vi "Unbundle.vi"(11 "Multi Instrument Wrapper Msg in":refnum<class "Multi Instrument Wrapper Msg.lvclass">) -> (0 "Aquirer Indices":i32[](array[numeric]), 1 "Aquirer":T1[](array[typedef]), 2 "Enqueue Locks":T2[](array[typedef]), 3 "Msg":refnum<class "Multi Instrument Msg.lvclass">)   [LabVIEW 2020, in "Instrument Handler.lvlib" / "Multi Instrument Wrapper Msg.lvclass"]
doc: "Unbundle all the private data from the Msg."
uses:
  Multi Instrument Wrapper Msg.lvclass
  Multi Instrument Msg/Multi Instrument Msg.lvclass
  Controls/Ctl_AquirerRefnum.ctl
  Multi Instrument Wrapper Msg.lvclass/Multi Instrument Wrapper Msg.ctl
  Instrument Handler.lvlib
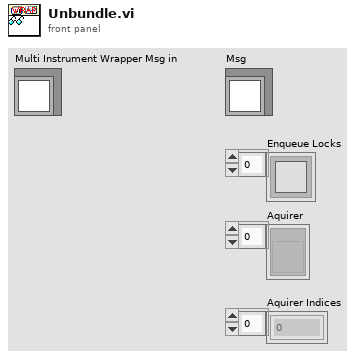
[diagram p1: front panel]
types:
  T1 = typedef "Instrument Handler.lvlib/Ctl_AquirerRefnum.ctl" = refnum<vi>
  T2 = typedef "Semaphore RefNum" = refnum<k1>
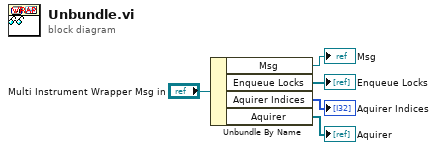
[diagram p0: block diagram]
diagram:
  n1 = Unbundle By Name("Multi Instrument Wrapper Msg in") -> ("Msg"=→"Msg":refnum<class "Multi Instrument Msg.lvclass">, "Enqueue Locks"=→"Enqueue Locks":T2[], "Aquirer Indices"=→"Aquirer Indices":i32[], "Aquirer"=→"Aquirer":T1[])
